vi "Generate Parameter JSON (array).vi"(6 "Replace Empty with 'null'":bool=TRUE, 9 "Value in Quotes":bool[](array[boolean]), 10 "Parameter Values":string[](array[string]), 11 "Parameter Names":string[](array[string])) -> (3 "Parameter Array JSON":string)   [LabVIEW 2015, in "NI_Azure_JSON Parsing.lvlib"]
uses:
  NI_Azure_JSON Parsing.lvlib
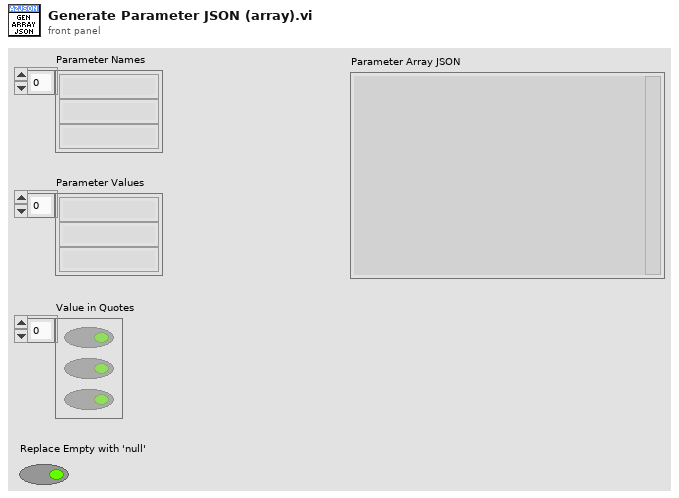
[diagram p1: front panel]
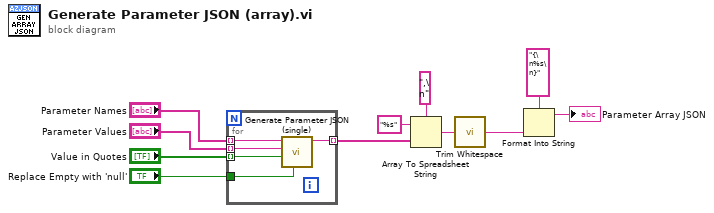
[diagram p0: block diagram]
diagram:
  n1 = for {
    tunnel: "Replace Empty with 'null'" -> [w16]
    tunnel: "Parameter Names" -> [w15] mode=indexing
    tunnel: "Parameter Values" -> [w14] mode=indexing
    tunnel: "Value in Quotes" -> [w13] mode=indexing
    tunnel: [w12] -> w9 mode=indexing
    n2 = call "Generate Parameter JSON (single).vi"("Replace Empty with 'null'"=w16, "Value in Quotes"=w13, "Parameter Value"=w14, "Parameter Name"=w15) -> ("Parameter JSON"=w12:string)  [unwired: 7 in]
  }
  n3 = Array To Spreadsheet String(delimiter (Tab)=",\n", array=w9, 3:"%s" ("format string")) -> (spreadsheet string=w6:string)
  n4 = call <vilib>:"Trim Whitespace.vi"("string"=w6) -> ("trimmed string"=w5:string)  [unwired: 1 in]
  n5 = Format Into String(format string="{\n%s\n}", w5) -> (resulting string=→"Parameter Array JSON":string)  [unwired: 2 in, 1 out]
